vi "ShowHideIncDec.vi"(8 "error in (no error)":errorcluster, 10 "Show?":bool, 11 "NumericRefs":refnum<vi>[](array[refnum])) -> (0 "error out":errorcluster, 3 "NumericRefs out":refnum<vi>[](array[refnum]))   [LabVIEW 2017, in "Align Elements.lvlib"]
uses:
  Align Elements.lvlib
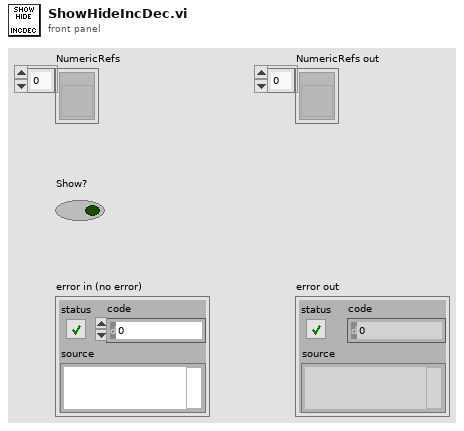
[diagram p1: front panel]
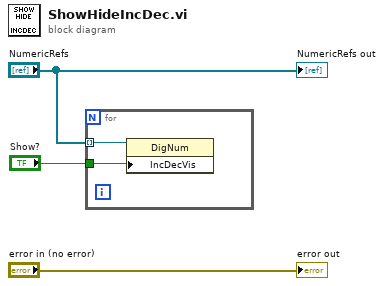
[diagram p0: block diagram]
diagram:
  n1 = for {
    tunnel: "NumericRefs" -> [w5] mode=indexing
    tunnel: "Show?" -> [w4]
    n2 = property class="DigNum"(reference=w5, "IncDecVis"=w4) -> ()  [unwired: 1 in, 2 out]
  }
  "NumericRefs out" <- "NumericRefs"
  "error out" <- "error in (no error)"
